vi "Unflatten UIP Value.vi"(10 "String Value":string, 11 "UIP In":refnum<class "SizeUIP.lvclass">) -> (0 "Error Out":errorcluster, 3 "UIP Out":refnum<class "SizeUIP.lvclass">)   [LabVIEW 2015, in "SizeUIP.lvclass"]
uses:
  SizeUIP.lvclass
  <vilib>/Utility/miscctls.llb/LVBoundsTypeDef.ctl
  SizeUIP.lvclass/SizeUIP.ctl
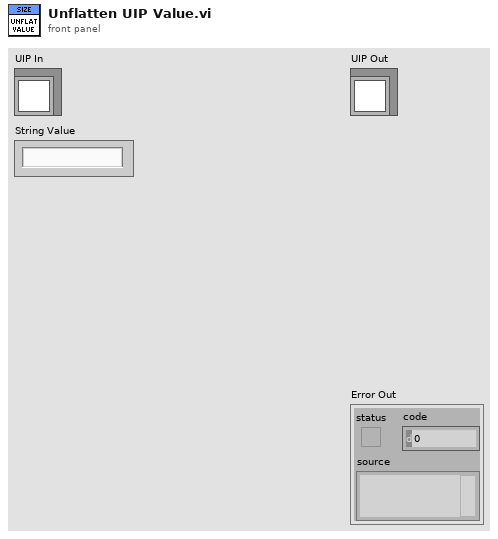
[diagram p1: front panel]
types:
  T1 = typedef "LVBoundsTypeDef.ctl" = cluster{"Width":u32, "Height":u32}
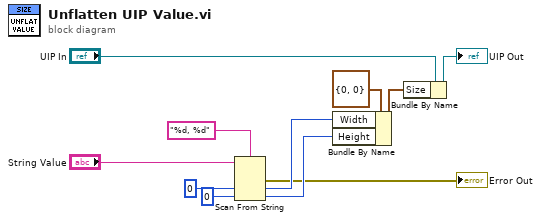
[diagram p0: block diagram]
diagram:
  n1 = Scan From String(format string="%d, %d", input string="String Value", default 1=u32 0, default 2=u32 0) -> (error out=→"Error Out":errorcluster, output 1=w6:u32, output 2=w5:u32)  [unwired: 2 in, 2 out]
  n2 = Bundle By Name(cluster=T1 {"Width"=0, "Height"=0} ("Size"), "Width"=w6, "Height"=w5) -> (w2:T1)
  n3 = Bundle By Name(cluster="UIP In", "Size"=w2) -> (→"UIP Out":refnum<class "SizeUIP.lvclass">)
